vi "Lab Panel V4.82.vi"() -> ()   [LabVIEW 2013] (continued)
                    n1780 = global write "Global 1.vi" "RATE(Hz)"("RATE (Hz)") -> ()
                    n1781 = global write "Global 1.vi" "SAMPLES"("SAMPLES") -> ()
                    n1782 = Index Array(array=w2725, index=6) -> (element=→"LAB04-1 (GRAPH)":dynamicdata)
                    n1783 = Index Array(array=w2725, index=7) -> (element=→"LAB04-2 (GRAPH)":dynamicdata)
                    n1784 = Index Array(array=w2725, index=9) -> (element=→"LAB05-2 (GRAPH)":dynamicdata)
                    n1785 = Index Array(array=w2725, index=8) -> (element=→"LAB05-1 (GRAPH)":dynamicdata)
                    n1786 = Index Array(array=w2725, index=5) -> (element=→"LAB03-2 (GRAPH)":dynamicdata)
                    n1787 = Index Array(array=w2725, index=0) -> (element=→"LAB01-1 (GRAPH)":dynamicdata)
                    n1788 = Index Array(array=w2725, index=1) -> (element=→"LAB01-2 (GRAPH)":dynamicdata)
                    n1789 = Index Array(array=w2725, index=2) -> (element=→"LAB02-1 (GRAPH)":dynamicdata)
                    n1790 = Index Array(array=w2725, index=3) -> (element=→"LAB02-2 (GRAPH)":dynamicdata)
                    n1791 = Index Array(array=w2725, index=4) -> (element=→"LAB03-1 (GRAPH)":dynamicdata)
                    "AI loop time" <- w2726
                    "Analog Error Array" <- w2727
                  }
                  frame #1 {
                    n1792 = Unbundle By Name(w2774) -> ("LAB05-1 (A)"=w2772:dbl, "LAB05-1 (V)"=w2771:dbl, "LAB05-1 (PF)"=w2770:dbl, "LAB05-2 (A)"=w2769:dbl, "LAB05-2 (V)"=w2768:dbl, "LAB05-2 (PF)"=w2767:dbl)
                    n1793 = case shown="False" w2750 {
                      tunnel: [w2775 w2776] -> w2773
                      tunnel: w2749 -> [_ w2776]
                      frame False {
                        n1794 = local read "CAL LAB01"() -> (w2775:T8)
                      }
                      frame True {
                      }
                    }
                    n1795 = Unbundle By Name(w2773) -> ("1  (A) cal"=w2766:dbl, "1 (V) cal"=w2765:dbl, "1 (PF) cal"=w2764:dbl, "2 (A) cal"=w2763:dbl, "2 (V) cal"=w2762:dbl, "2 (PF) cal"=w2761:dbl)  [unwired: 4 out]
                    n1796 = Multiply(x=w2772, y=w2766) -> (x*y=w2759:dbl)
                    n1797 = Multiply(x=w2771, y=w2765) -> (x*y=w2758:dbl)
                    n1798 = Multiply(x=w2770, y=w2764) -> (x*y=w2757:dbl)
                    n1799 = Multiply(x=w2769, y=w2763) -> (x*y=w2753:dbl)
                    n1800 = Multiply(x=w2768, y=w2762) -> (x*y=w2752:dbl)
                    n1801 = Multiply(x=w2767, y=w2761) -> (x*y=w2751:dbl)
                    n1802 = local read "SIG LAB01-1"() -> (w2760:T2)
                    n1803 = local read "SIG LAB01-2"() -> (w2755:T2)
                    n1804 = Bundle By Name(cluster=w2760, "AMPS"=w2759, "VOLTS"=w2758, "PF"=w2757) -> (w2756:T2)
                    n1805 = Bundle By Name(cluster=w2755, "AMPS"=w2753, "VOLTS"=w2752, "PF"=w2751) -> (w2754:T2)
                    n1806 = local write "SIG LAB01-2"(w2754) -> ()
                    n1807 = local write "SIG LAB01-1"(w2756) -> ()
                  }
                  frame #2 {
                    n1808 = Unbundle By Name(w2779) -> ("LAB05-1 (A)"=w2801:dbl, "LAB05-1 (V)"=w2800:dbl, "LAB05-1 (PF)"=w2799:dbl, "LAB05-2 (A)"=w2798:dbl, "LAB05-2 (V)"=w2797:dbl, "LAB05-2 (PF)"=w2796:dbl)
                    n1809 = case shown="True" w2778 {
                      tunnel: [w2803 w2804] -> w2802
                      tunnel: w2777 -> [_ w2804]
                      frame False {
                        n1810 = local read "CAL LAB02"() -> (w2803:T9)
                      }
                      frame True {
                      }
                    }
                    n1811 = Unbundle By Name(w2802) -> ("1  (A) cal"=w2795:dbl, "1 (V) cal"=w2794:dbl, "1 (PF) cal"=w2793:dbl, "2 (A) cal"=w2792:dbl, "2 (V) cal"=w2791:dbl, "2 (PF) cal"=w2790:dbl)  [unwired: 4 out]
                    n1812 = Multiply(x=w2801, y=w2795) -> (x*y=w2788:dbl)
                    n1813 = Multiply(x=w2800, y=w2794) -> (x*y=w2787:dbl)
                    n1814 = Multiply(x=w2799, y=w2793) -> (x*y=w2786:dbl)
                    n1815 = Multiply(x=w2798, y=w2792) -> (x*y=w2782:dbl)
                    n1816 = Multiply(x=w2797, y=w2791) -> (x*y=w2781:dbl)
                    n1817 = Multiply(x=w2796, y=w2790) -> (x*y=w2780:dbl)
                    n1818 = local read "SIG LAB02-1"() -> (w2789:T2)
                    n1819 = local read "SIG LAB02-2"() -> (w2784:T2)
                    n1820 = Bundle By Name(cluster=w2789, "AMPS"=w2788, "VOLTS"=w2787, "PF"=w2786) -> (w2785:T2)
                    n1821 = Bundle By Name(cluster=w2784, "AMPS"=w2782, "VOLTS"=w2781, "PF"=w2780) -> (w2783:T2)
                    n1822 = local write "SIG LAB02-2"(w2783) -> ()
                    n1823 = local write "SIG LAB02-1"(w2785) -> ()
                  }
                  frame #3 {
                    n1824 = Unbundle By Name(w2808) -> ("LAB05-1 (A)"=w2829:dbl, "LAB05-1 (V)"=w2828:dbl, "LAB05-1 (PF)"=w2827:dbl, "LAB05-2 (A)"=w2826:dbl, "LAB05-2 (V)"=w2825:dbl, "LAB05-2 (PF)"=w2824:dbl)
                    n1825 = case shown="True" w2806 {
                      tunnel: [w2831 w2832] -> w2830
                      tunnel: w2805 -> [_ w2832]
                      frame False {
                        n1826 = local read "CAL LAB03"() -> (w2831:T8)
                      }
                      frame True {
                      }
                    }
                    n1827 = Unbundle By Name(w2830) -> ("1  (A) cal"=w2823:dbl, "1 (V) cal"=w2822:dbl, "1 (PF) cal"=w2821:dbl, "2 (A) cal"=w2820:dbl, "2 (V) cal"=w2819:dbl, "2 (PF) cal"=w2818:dbl)  [unwired: 4 out]
                    n1828 = Multiply(x=w2829, y=w2823) -> (x*y=w2816:dbl)
                    n1829 = Multiply(x=w2828, y=w2822) -> (x*y=w2807:dbl)
                    n1830 = Multiply(x=w2827, y=w2821) -> (x*y=w2815:dbl)
                    n1831 = Multiply(x=w2826, y=w2820) -> (x*y=w2811:dbl)
                    n1832 = Multiply(x=w2825, y=w2819) -> (x*y=w2810:dbl)
                    n1833 = Multiply(x=w2824, y=w2818) -> (x*y=w2809:dbl)
                    n1834 = local read "SIG LAB03-1"() -> (w2817:T2)
                    n1835 = local read "SIG LAB03-2"() -> (w2813:T2)
                    n1836 = Bundle By Name(cluster=w2817, "AMPS"=w2816, "VOLTS"=w2807, "PF"=w2815) -> (w2814:T2)
                    n1837 = Bundle By Name(cluster=w2813, "AMPS"=w2811, "VOLTS"=w2810, "PF"=w2809) -> (w2812:T2)
                    n1838 = local write "SIG LAB03-2"(w2812) -> ()
                    n1839 = local write "SIG LAB03-1"(w2814) -> ()
                  }
                  frame #4 {
                    n1840 = Unbundle By Name(w2835) -> ("LAB05-1 (A)"=w2857:dbl, "LAB05-1 (V)"=w2856:dbl, "LAB05-1 (PF)"=w2855:dbl, "LAB05-2 (A)"=w2854:dbl, "LAB05-2 (V)"=w2853:dbl, "LAB05-2 (PF)"=w2852:dbl)
                    n1841 = case shown="False" w2834 {
                      tunnel: [w2859 w2860] -> w2858
                      tunnel: w2833 -> [_ w2860]
                      frame False {
                        n1842 = local read "CAL LAB04"() -> (w2859:T8)
                      }
                      frame True {
                      }
                    }
                    n1843 = Unbundle By Name(w2858) -> ("1  (A) cal"=w2851:dbl, "1 (V) cal"=w2850:dbl, "1 (PF) cal"=w2849:dbl, "2 (A) cal"=w2848:dbl, "2 (V) cal"=w2847:dbl, "2 (PF) cal"=w2846:dbl)  [unwired: 4 out]
                    n1844 = Multiply(x=w2857, y=w2851) -> (x*y=w2844:dbl)
                    n1845 = Multiply(x=w2856, y=w2850) -> (x*y=w2843:dbl)
                    n1846 = Multiply(x=w2855, y=w2849) -> (x*y=w2842:dbl)
                    n1847 = Multiply(x=w2854, y=w2848) -> (x*y=w2838:dbl)
                    n1848 = Multiply(x=w2853, y=w2847) -> (x*y=w2837:dbl)
                    n1849 = Multiply(x=w2852, y=w2846) -> (x*y=w2836:dbl)
                    n1850 = local read "SIG LAB04-1"() -> (w2845:T2)
                    n1851 = local read "SIG LAB04-2"() -> (w2840:T2)
                    n1852 = Bundle By Name(cluster=w2845, "AMPS"=w2844, "VOLTS"=w2843, "PF"=w2842) -> (w2841:T2)
                    n1853 = Bundle By Name(cluster=w2840, "AMPS"=w2838, "VOLTS"=w2837, "PF"=w2836) -> (w2839:T2)
                    n1854 = local write "SIG LAB04-2"(w2839) -> ()
                    n1855 = local write "SIG LAB04-1"(w2841) -> ()
                  }
                  frame #5 {
                    n1856 = Unbundle By Name(w2864) -> ("LAB05-1 (A)"=w2885:dbl, "LAB05-1 (V)"=w2863:dbl, "LAB05-1 (PF)"=w2884:dbl, "LAB05-2 (A)"=w2883:dbl, "LAB05-2 (V)"=w2882:dbl, "LAB05-2 (PF)"=w2881:dbl)
                    n1857 = case shown="False" w2862 {
                      tunnel: [w2887 w2888] -> w2886
                      tunnel: w2861 -> [_ w2888]
                      frame False {
                        n1858 = local read "CAL LAB05"() -> (w2887:T8)
                      }
                      frame True {
                      }
                    }
                    n1859 = Unbundle By Name(w2886) -> ("1  (A) cal"=w2880:dbl, "1 (V) cal"=w2879:dbl, "1 (PF) cal"=w2878:dbl, "2 (A) cal"=w2877:dbl, "2 (V) cal"=w2876:dbl, "2 (PF) cal"=w2875:dbl)  [unwired: 4 out]
                    n1860 = Multiply(x=w2885, y=w2880) -> (x*y=w2873:dbl)
                    n1861 = Multiply(x=w2863, y=w2879) -> (x*y=w2872:dbl)
                    n1862 = Multiply(x=w2884, y=w2878) -> (x*y=w2871:dbl)
                    n1863 = Multiply(x=w2883, y=w2877) -> (x*y=w2867:dbl)
                    n1864 = Multiply(x=w2882, y=w2876) -> (x*y=w2866:dbl)
                    n1865 = Multiply(x=w2881, y=w2875) -> (x*y=w2865:dbl)
                    n1866 = local read "SIG LAB05-1"() -> (w2874:T2)
                    n1867 = local read "SIG LAB05-2"() -> (w2869:T2)
                    n1868 = Bundle By Name(cluster=w2874, "AMPS"=w2873, "VOLTS"=w2872, "PF"=w2871) -> (w2870:T2)
                    n1869 = Bundle By Name(cluster=w2869, "AMPS"=w2867, "VOLTS"=w2866, "PF"=w2865) -> (w2868:T2)
                    n1870 = local write "SIG LAB05-2"(w2868) -> ()
                    n1871 = local write "SIG LAB05-1"(w2870) -> ()
                  }
                }
              }
            }
          }
          frame #12 {
            # "save test data to file"
            n1872 = Get Date/Time In Seconds() -> (seconds since 1Jan1904=w2889:timestamp)
            "File Time Stamp" <- w2889
            n1873 = local read "on loops"() -> (w2908:dbl)
            n1874 = local read "jig cycle"() -> (w2905:dbl)
            n1875 = Format Date/Time String(time format string (%c)="%H:%M%:%S", seconds (now)=w2889) -> (date/time string=w2893:string)  [unwired: 1 in]
            n1876 = Add(x=w2908, y=2) -> (x+y=w2906:dbl)
            n1877 = Build Array(w2893) -> (w2892:string[])
            n1878 = Equal?(x=w2905, y=1) -> (x = y?=w2891:bool)
            n1879 = Equal?(x=w2905, y=w2906) -> (x = y?=w2890:bool)
            n1880 = stacked-sequence {
              tunnel: w2904 -> [w2914 _ _ _ _ _ _ _ _ _]
              tunnel: w2903 -> [_ w2990 _ _ _ _ _ _ _ _]
              tunnel: w2902 -> [_ _ w3070 _ _ _ _ _ _ _]
              tunnel: w2901 -> [_ _ _ w3150 _ _ _ _ _ _]
              tunnel: w2900 -> [_ _ _ _ w3230 _ _ _ _ _]
              tunnel: w2899 -> [_ _ _ _ _ w3310 _ _ _ _]
              tunnel: w2898 -> [_ _ _ _ _ _ w3390 _ _ _]
              tunnel: w2897 -> [_ _ _ _ _ _ _ w3470 _ _]
              tunnel: w2896 -> [_ _ _ _ _ _ _ _ w3550 _]
              tunnel: w2895 -> [_ _ _ _ _ _ _ _ _ w3630]
              tunnel: w2892 -> [w2913 w2994 w3074 w3154 w3234 w3314 w3394 w3474 w3554 w3634]
              tunnel: w2891 -> [w2912 w2993 w3073 w3153 w3233 w3313 w3393 w3473 w3553 w3633]
              tunnel: w2890 -> [w2911 w2992 w3072 w3152 w3232 w3312 w3392 w3472 w3552 w3632]
              tunnel: w2889 -> [w2910 w2991 w3071 w3151 w3231 w3311 w3391 w3471 w3551 w3631]
              frame #0 {
                n1881 = case shown="True" w2914 {
                  tunnel: w2913 -> [_ w2919]
                  tunnel: w2912 -> [_ w2918]
                  tunnel: w2911 -> [_ w2916]
                  tunnel: w2910 -> [_ w2915]
                  frame False {
                  }
                  frame True {
                    n1882 = local read "DISP LAB01-1"() -> (w2920:T4)
                    n1883 = local read "SIG LAB01-1"() -> (w2921:T2)
                    n1884 = local read "ON L01-1"() -> (w2917:cluster{"amps":dbl, "volts":dbl, "pf":dbl})
                    n1885 = Unbundle(w2921) -> ("AMPS"=w2927:dbl, "VOLTS"=w2925:dbl, "PF"=w2924:dbl, "Tmp Live"=w2923:dbl, "Tmp Neut"=w2926:dbl)
                    n1886 = Unbundle(w2920) -> ("CYCLE"=w2922:dbl)  [unwired: 2 out]
                    n1887 = stacked-sequence {
                      tunnel: w2927 -> [w2931 w2950]
                      tunnel: w2926 -> [_ w2949]
                      tunnel: w2925 -> [w2930 w2948]
                      tunnel: w2924 -> [w2929 w2947]
                      tunnel: w2923 -> [_ w2946]
                      tunnel: w2922 -> [_ w2945]
                      tunnel: w2919 -> [_ w2944]
                      tunnel: w2918 -> [w2932 _]
                      tunnel: w2917 -> [w2928 w2942]
                      tunnel: w2916 -> [_ w2943]
                      tunnel: w2915 -> [_ w2938]
                      frame #0 {
                        n1888 = case shown="True" w2932 {
                          tunnel: w2931 -> [_ w2937]
                          tunnel: w2930 -> [_ w2936]
                          tunnel: w2929 -> [_ w2935]
                          tunnel: w2928 -> [_ w2933]
                          frame False {
                          }
                          frame True {
                            n1889 = Bundle(cluster=w2933, "amps"=w2937, "volts"=w2936, "pf"=w2935) -> (w2934:cluster{"amps":dbl, "volts":dbl, "pf":dbl})
                            n1890 = local write "ON L01-1"(w2934) -> ()
                          }
                        }
                      }
                      frame #1 {
                        n1891 = Unbundle(w2942) -> ("amps"=w2941:dbl, "volts"=w2940:dbl, "pf"=w2939:dbl)
                        n1892 = case shown="True" w2943 {
                          tunnel: w2950 -> [_ w2951]
                          tunnel: w2949 -> [_ w2989]
                          tunnel: w2948 -> [_ _]
                          tunnel: w2947 -> [_ _]
                          tunnel: w2946 -> [_ w2988]
                          tunnel: w2945 -> [_ w2987]
                          tunnel: w2944 -> [_ w2955]
                          tunnel: w2941 -> [_ w2952]
                          tunnel: w2940 -> [_ w2984]
                          tunnel: w2939 -> [_ w2983]
                          tunnel: w2938 -> [_ w2953]
                          frame False {
                          }
                          frame True {
                            n1893 = local read "TDMS LAB01-1"() -> (w2986:refnum<k34>)
                            n1894 = Build Array(w2984) -> (w2980:dbl[])
                            n1895 = Build Array(w2983) -> (w2979:dbl[])
                            n1896 = Build Array(w2988) -> (w2978:dbl[])
                            n1897 = Build Array(w2989) -> (w2977:dbl[])
                            n1898 = Build Array(w2952) -> (w2982:dbl[])
                            n1899 = Build Array(w2951) -> (w2981:dbl[])
                            n1900 = Build Array(w2987) -> (w2976:dbl[])
                            n1901 = Build Array("AMPS ON", "AMPS OFF", "VOLTS", "PF", "TEMP Live", "TEMP Neut", "CYCLE") -> (w2960:string[])
                            n1902 = Bundle By Name("Y"=w2982, "t0"=w2953) -> (w2975:waveform(dbl))  [unwired: 1 in]
                            n1903 = Bundle By Name("Y"=w2981, "t0"=w2953) -> (w2974:waveform(dbl))  [unwired: 1 in]
                            n1904 = Bundle By Name("Y"=w2980, "t0"=w2953) -> (w2973:waveform(dbl))  [unwired: 1 in]
                            n1905 = Bundle By Name("Y"=w2979, "t0"=w2953) -> (w2972:waveform(dbl))  [unwired: 1 in]
                            n1906 = Bundle By Name("Y"=w2978, "t0"=w2953) -> (w2971:waveform(dbl))  [unwired: 1 in]
                            n1907 = Bundle By Name("Y"=w2977, "t0"=w2953) -> (w2970:waveform(dbl))  [unwired: 1 in]
                            n1908 = Bundle By Name("Y"=w2976, "t0"=w2953) -> (w2969:waveform(dbl))  [unwired: 1 in]
                            n1909 = Build Array(w2975, w2974, w2973, w2972, w2971, w2970, w2969) -> (w2968:waveform(dbl)[])
                            n1910 = TDMS Write(0:w2986, 5:"TEST VALUES", 7:w2960, 9:w2968) -> (4:w2959:refnum<k34>, 6:w2958:string, 15:w2957:errorcluster)  [unwired: 2 in, 1 out]
                            n1911 = TDMS Write(0:w2959, 5:w2958, 7:"TIME", 9:w2955, 11:w2957) -> (15:w2954:errorcluster)  [unwired: 1 in, 3 out]
                            n1912 = local write "data file error"(w2954) -> ()
                          }
                        }
                      }
                    }
                  }
                }
              }
              frame #1 {
                n1913 = case shown="True" w2990 {
                  tunnel: w2994 -> [_ w2999]
                  tunnel: w2993 -> [_ w2998]
                  tunnel: w2992 -> [_ w2996]
                  tunnel: w2991 -> [_ w2995]
                  frame False {
                  }
                  frame True {
                    n1914 = local read "DISP LAB01-2"() -> (w3000:T4)
                    n1915 = local read "SIG LAB01-2"() -> (w3001:T2)
                    n1916 = local read "ON L01-2"() -> (w2997:cluster{"amps":dbl, "volts":dbl, "pf":dbl})
                    n1917 = Unbundle(w3001) -> ("AMPS"=w3007:dbl, "VOLTS"=w3005:dbl, "PF"=w3004:dbl, "Tmp Live"=w3003:dbl, "Tmp Neut"=w3006:dbl)
                    n1918 = Unbundle(w3000) -> ("CYCLE"=w3002:dbl)  [unwired: 2 out]
                    n1919 = stacked-sequence {
                      tunnel: w3007 -> [w3011 w3030]
                      tunnel: w3006 -> [_ w3029]
                      tunnel: w3005 -> [w3010 w3028]
                      tunnel: w3004 -> [w3009 w3027]
                      tunnel: w3003 -> [_ w3026]
                      tunnel: w3002 -> [_ w3025]
                      tunnel: w2999 -> [_ w3024]
                      tunnel: w2998 -> [w3012 _]
                      tunnel: w2997 -> [w3008 w3022]
                      tunnel: w2996 -> [_ w3023]
                      tunnel: w2995 -> [_ w3018]
                      frame #0 {
                        n1920 = case shown="True" w3012 {
                          tunnel: w3011 -> [_ w3017]
                          tunnel: w3010 -> [_ w3016]
                          tunnel: w3009 -> [_ w3015]
                          tunnel: w3008 -> [_ w3013]
                          frame False {
                          }
                          frame True {
                            n1921 = Bundle(cluster=w3013, "amps"=w3017, "volts"=w3016, "pf"=w3015) -> (w3014:cluster{"amps":dbl, "volts":dbl, "pf":dbl})
                            n1922 = local write "ON L01-2"(w3014) -> ()
                          }
                        }
                      }
                      frame #1 {
                        n1923 = Unbundle(w3022) -> ("amps"=w3021:dbl, "volts"=w3020:dbl, "pf"=w3019:dbl)
                        n1924 = case shown="True" w3023 {
                          tunnel: w3030 -> [_ w3062]
                          tunnel: w3029 -> [_ w3069]
                          tunnel: w3028 -> [_ _]
                          tunnel: w3027 -> [_ _]
                          tunnel: w3026 -> [_ w3068]
                          tunnel: w3025 -> [_ w3067]
                          tunnel: w3024 -> [_ w3032]
                          tunnel: w3021 -> [_ w3064]
                          tunnel: w3020 -> [_ w3063]
                          tunnel: w3019 -> [_ w3061]
                          tunnel: w3018 -> [_ w3053]
                          frame False {
                          }
                          frame True {
                            n1925 = local read "TDMS LAB01-2"() -> (w3066:refnum<k34>)
                            n1926 = Build Array(w3063) -> (w3058:dbl[])
                            n1927 = Build Array(w3061) -> (w3057:dbl[])
                            n1928 = Build Array(w3068) -> (w3056:dbl[])
                            n1929 = Build Array(w3069) -> (w3055:dbl[])
                            n1930 = Build Array(w3064) -> (w3060:dbl[])
                            n1931 = Build Array(w3062) -> (w3059:dbl[])
                            n1932 = Build Array(w3067) -> (w3054:dbl[])
                            n1933 = Build Array("AMPS ON", "AMPS OFF", "VOLTS", "PF", "TEMP Live", "TEMP Neut", "CYCLE") -> (w3037:string[])
                            n1934 = Bundle By Name("Y"=w3060, "t0"=w3053) -> (w3052:waveform(dbl))  [unwired: 1 in]
                            n1935 = Bundle By Name("Y"=w3059, "t0"=w3053) -> (w3051:waveform(dbl))  [unwired: 1 in]
                            n1936 = Bundle By Name("Y"=w3058, "t0"=w3053) -> (w3050:waveform(dbl))  [unwired: 1 in]
                            n1937 = Bundle By Name("Y"=w3057, "t0"=w3053) -> (w3049:waveform(dbl))  [unwired: 1 in]
                            n1938 = Bundle By Name("Y"=w3056, "t0"=w3053) -> (w3048:waveform(dbl))  [unwired: 1 in]
                            n1939 = Bundle By Name("Y"=w3055, "t0"=w3053) -> (w3047:waveform(dbl))  [unwired: 1 in]
                            n1940 = Bundle By Name("Y"=w3054, "t0"=w3053) -> (w3046:waveform(dbl))  [unwired: 1 in]
                            n1941 = Build Array(w3052, w3051, w3050, w3049, w3048, w3047, w3046) -> (w3045:waveform(dbl)[])
                            n1942 = TDMS Write(0:w3066, 5:"TEST VALUES", 7:w3037, 9:w3045) -> (4:w3036:refnum<k34>, 6:w3035:string, 15:w3034:errorcluster)  [unwired: 2 in, 1 out]
                            n1943 = TDMS Write(0:w3036, 5:w3035, 7:"TIME", 9:w3032, 11:w3034) -> (15:w3031:errorcluster)  [unwired: 1 in, 3 out]
                            n1944 = local write "data file error"(w3031) -> ()
                          }
                        }
                      }
                    }
                  }
                }
              }
              frame #2 {
                n1945 = case shown="True" w3070 {
                  tunnel: w3074 -> [_ w3079]
                  tunnel: w3073 -> [_ w3078]
                  tunnel: w3072 -> [_ w3076]
                  tunnel: w3071 -> [_ w3075]
                  frame False {
                  }
                  frame True {
                    n1946 = local read "DISP LAB02-1"() -> (w3080:T4)
                    n1947 = local read "SIG LAB02-1"() -> (w3081:T2)
                    n1948 = local read "ON L02-1"() -> (w3077:cluster{"amps":dbl, "volts":dbl, "pf":dbl})
                    n1949 = Unbundle(w3081) -> ("AMPS"=w3087:dbl, "VOLTS"=w3085:dbl, "PF"=w3084:dbl, "Tmp Live"=w3083:dbl, "Tmp Neut"=w3086:dbl)
                    n1950 = Unbundle(w3080) -> ("CYCLE"=w3082:dbl)  [unwired: 2 out]
                    n1951 = stacked-sequence {
                      tunnel: w3087 -> [w3091 w3110]
                      tunnel: w3086 -> [_ w3109]
                      tunnel: w3085 -> [w3090 w3108]
                      tunnel: w3084 -> [w3089 w3107]
                      tunnel: w3083 -> [_ w3106]
                      tunnel: w3082 -> [_ w3105]
                      tunnel: w3079 -> [_ w3104]
                      tunnel: w3078 -> [w3092 _]
                      tunnel: w3077 -> [w3088 w3102]
                      tunnel: w3076 -> [_ w3103]
                      tunnel: w3075 -> [_ w3098]
                      frame #0 {
                        n1952 = case shown="True" w3092 {
                          tunnel: w3091 -> [_ w3097]
                          tunnel: w3090 -> [_ w3096]
                          tunnel: w3089 -> [_ w3095]
                          tunnel: w3088 -> [_ w3093]
                          frame False {
                          }
                          frame True {
                            n1953 = Bundle(cluster=w3093, "amps"=w3097, "volts"=w3096, "pf"=w3095) -> (w3094:cluster{"amps":dbl, "volts":dbl, "pf":dbl})
                            n1954 = local write "ON L02-1"(w3094) -> ()
                          }
                        }
                      }
                      frame #1 {
                        n1955 = Unbundle(w3102) -> ("amps"=w3101:dbl, "volts"=w3100:dbl, "pf"=w3099:dbl)
                        n1956 = case shown="True" w3103 {
                          tunnel: w3110 -> [_ w3142]
                          tunnel: w3109 -> [_ w3149]
                          tunnel: w3108 -> [_ _]
                          tunnel: w3107 -> [_ _]
                          tunnel: w3106 -> [_ w3148]
                          tunnel: w3105 -> [_ w3147]
                          tunnel: w3104 -> [_ w3112]
                          tunnel: w3101 -> [_ w3144]
                          tunnel: w3100 -> [_ w3143]
                          tunnel: w3099 -> [_ w3141]
                          tunnel: w3098 -> [_ w3133]
                          frame False {
                          }
                          frame True {
                            n1957 = local read "TDMS LAB02-1"() -> (w3146:refnum<k34>)
                            n1958 = Build Array(w3143) -> (w3138:dbl[])
                            n1959 = Build Array(w3141) -> (w3137:dbl[])
                            n1960 = Build Array(w3148) -> (w3136:dbl[])
                            n1961 = Build Array(w3149) -> (w3135:dbl[])
                            n1962 = Build Array(w3144) -> (w3140:dbl[])
                            n1963 = Build Array(w3142) -> (w3139:dbl[])
                            n1964 = Build Array(w3147) -> (w3134:dbl[])
                            n1965 = Build Array("AMPS ON", "AMPS OFF", "VOLTS", "PF", "TEMP Live", "TEMP Neut", "CYCLE") -> (w3117:string[])
                            n1966 = Bundle By Name("Y"=w3140, "t0"=w3133) -> (w3132:waveform(dbl))  [unwired: 1 in]
                            n1967 = Bundle By Name("Y"=w3139, "t0"=w3133) -> (w3131:waveform(dbl))  [unwired: 1 in]
                            n1968 = Bundle By Name("Y"=w3138, "t0"=w3133) -> (w3130:waveform(dbl))  [unwired: 1 in]
                            n1969 = Bundle By Name("Y"=w3137, "t0"=w3133) -> (w3129:waveform(dbl))  [unwired: 1 in]
                            n1970 = Bundle By Name("Y"=w3136, "t0"=w3133) -> (w3128:waveform(dbl))  [unwired: 1 in]
                            n1971 = Bundle By Name("Y"=w3135, "t0"=w3133) -> (w3127:waveform(dbl))  [unwired: 1 in]
                            n1972 = Bundle By Name("Y"=w3134, "t0"=w3133) -> (w3126:waveform(dbl))  [unwired: 1 in]
                            n1973 = Build Array(w3132, w3131, w3130, w3129, w3128, w3127, w3126) -> (w3125:waveform(dbl)[])
                            n1974 = TDMS Write(0:w3146, 5:"TEST VALUES", 7:w3117, 9:w3125) -> (4:w3116:refnum<k34>, 6:w3115:string, 15:w3114:errorcluster)  [unwired: 2 in, 1 out]
                            n1975 = TDMS Write(0:w3116, 5:w3115, 7:"TIME", 9:w3112, 11:w3114) -> (15:w3111:errorcluster)  [unwired: 1 in, 3 out]
                            n1976 = local write "data file error"(w3111) -> ()
                          }
                        }
                      }
                    }
                  }
                }
              }
              frame #3 {
                n1977 = case shown="True" w3150 {
                  tunnel: w3154 -> [_ w3159]
                  tunnel: w3153 -> [_ w3158]
                  tunnel: w3152 -> [_ w3156]
                  tunnel: w3151 -> [_ w3155]
                  frame False {
                  }
                  frame True {
                    n1978 = local read "DISP LAB02-2"() -> (w3160:T4)
                    n1979 = local read "SIG LAB02-2"() -> (w3161:T2)
                    n1980 = local read "ON L02-2"() -> (w3157:cluster{"amps":dbl, "volts":dbl, "pf":dbl})
                    n1981 = Unbundle(w3161) -> ("AMPS"=w3167:dbl, "VOLTS"=w3165:dbl, "PF"=w3164:dbl, "Tmp Live"=w3163:dbl, "Tmp Neut"=w3166:dbl)
                    n1982 = Unbundle(w3160) -> ("CYCLE"=w3162:dbl)  [unwired: 2 out]
                    n1983 = stacked-sequence {
                      tunnel: w3167 -> [w3171 w3190]
                      tunnel: w3166 -> [_ w3189]
                      tunnel: w3165 -> [w3170 w3188]
                      tunnel: w3164 -> [w3169 w3187]
                      tunnel: w3163 -> [_ w3186]
                      tunnel: w3162 -> [_ w3185]
                      tunnel: w3159 -> [_ w3184]
                      tunnel: w3158 -> [w3172 _]
                      tunnel: w3157 -> [w3168 w3182]
                      tunnel: w3156 -> [_ w3183]
                      tunnel: w3155 -> [_ w3178]
                      frame #0 {
                        n1984 = case shown="True" w3172 {
                          tunnel: w3171 -> [_ w3177]
                          tunnel: w3170 -> [_ w3176]
                          tunnel: w3169 -> [_ w3175]
                          tunnel: w3168 -> [_ w3173]
                          frame False {
                          }
                          frame True {
                            n1985 = Bundle(cluster=w3173, "amps"=w3177, "volts"=w3176, "pf"=w3175) -> (w3174:cluster{"amps":dbl, "volts":dbl, "pf":dbl})
                            n1986 = local write "ON L02-2"(w3174) -> ()
                          }
                        }
                      }
                      frame #1 {
                        n1987 = Unbundle(w3182) -> ("amps"=w3181:dbl, "volts"=w3180:dbl, "pf"=w3179:dbl)
                        n1988 = case shown="True" w3183 {
                          tunnel: w3190 -> [_ w3222]
                          tunnel: w3189 -> [_ w3229]
                          tunnel: w3188 -> [_ _]
                          tunnel: w3187 -> [_ _]
                          tunnel: w3186 -> [_ w3228]
                          tunnel: w3185 -> [_ w3227]
                          tunnel: w3184 -> [_ w3192]
                          tunnel: w3181 -> [_ w3224]
                          tunnel: w3180 -> [_ w3223]
                          tunnel: w3179 -> [_ w3221]
                          tunnel: w3178 -> [_ w3213]
                          frame False {
                          }
                          frame True {
                            n1989 = local read "TDMS LAB02-2"() -> (w3226:refnum<k34>)
                            n1990 = Build Array(w3223) -> (w3218:dbl[])
                            n1991 = Build Array(w3221) -> (w3217:dbl[])
                            n1992 = Build Array(w3228) -> (w3216:dbl[])
                            n1993 = Build Array(w3229) -> (w3215:dbl[])
                            n1994 = Build Array(w3224) -> (w3220:dbl[])
                            n1995 = Build Array(w3222) -> (w3219:dbl[])
                            n1996 = Build Array(w3227) -> (w3214:dbl[])
                            n1997 = Build Array("AMPS ON", "AMPS OFF", "VOLTS", "PF", "TEMP Live", "TEMP Neut", "CYCLE") -> (w3197:string[])
                            n1998 = Bundle By Name("Y"=w3220, "t0"=w3213) -> (w3212:waveform(dbl))  [unwired: 1 in]
                            n1999 = Bundle By Name("Y"=w3219, "t0"=w3213) -> (w3211:waveform(dbl))  [unwired: 1 in]
                            n2000 = Bundle By Name("Y"=w3218, "t0"=w3213) -> (w3210:waveform(dbl))  [unwired: 1 in]
                            n2001 = Bundle By Name("Y"=w3217, "t0"=w3213) -> (w3209:waveform(dbl))  [unwired: 1 in]
                            n2002 = Bundle By Name("Y"=w3216, "t0"=w3213) -> (w3208:waveform(dbl))  [unwired: 1 in]
                            n2003 = Bundle By Name("Y"=w3215, "t0"=w3213) -> (w3207:waveform(dbl))  [unwired: 1 in]
                            n2004 = Bundle By Name("Y"=w3214, "t0"=w3213) -> (w3206:waveform(dbl))  [unwired: 1 in]
                            n2005 = Build Array(w3212, w3211, w3210, w3209, w3208, w3207, w3206) -> (w3205:waveform(dbl)[])
                            n2006 = TDMS Write(0:w3226, 5:"TEST VALUES", 7:w3197, 9:w3205) -> (4:w3196:refnum<k34>, 6:w3195:string, 15:w3194:errorcluster)  [unwired: 2 in, 1 out]
                            n2007 = TDMS Write(0:w3196, 5:w3195, 7:"TIME", 9:w3192, 11:w3194) -> (15:w3191:errorcluster)  [unwired: 1 in, 3 out]
                            n2008 = local write "data file error"(w3191) -> ()
                          }
                        }
                      }
                    }
                  }
                }
              }
              frame #4 {
                n2009 = case shown="True" w3230 {
                  tunnel: w3234 -> [_ w3239]
                  tunnel: w3233 -> [_ w3238]
                  tunnel: w3232 -> [_ w3236]
                  tunnel: w3231 -> [_ w3235]
                  frame False {
                  }
                  frame True {
                    n2010 = local read "DISP LAB03-1"() -> (w3240:T4)
                    n2011 = local read "SIG LAB03-1"() -> (w3241:T2)
                    n2012 = local read "ON L03-1"() -> (w3237:cluster{"amps":dbl, "volts":dbl, "pf":dbl})
                    n2013 = Unbundle(w3241) -> ("AMPS"=w3247:dbl, "VOLTS"=w3245:dbl, "PF"=w3244:dbl, "Tmp Live"=w3243:dbl, "Tmp Neut"=w3246:dbl)
                    n2014 = Unbundle(w3240) -> ("CYCLE"=w3242:dbl)  [unwired: 2 out]
                    n2015 = stacked-sequence {
                      tunnel: w3247 -> [w3251 w3270]
                      tunnel: w3246 -> [_ w3269]
                      tunnel: w3245 -> [w3250 w3268]
                      tunnel: w3244 -> [w3249 w3267]
                      tunnel: w3243 -> [_ w3266]
                      tunnel: w3242 -> [_ w3265]
                      tunnel: w3239 -> [_ w3264]
                      tunnel: w3238 -> [w3252 _]
                      tunnel: w3237 -> [w3248 w3262]
                      tunnel: w3236 -> [_ w3263]
                      tunnel: w3235 -> [_ w3258]
                      frame #0 {
                        n2016 = case shown="True" w3252 {
                          tunnel: w3251 -> [_ w3257]
                          tunnel: w3250 -> [_ w3256]
                          tunnel: w3249 -> [_ w3255]
                          tunnel: w3248 -> [_ w3253]
                          frame False {
                          }
                          frame True {
                            n2017 = Bundle(cluster=w3253, "amps"=w3257, "volts"=w3256, "pf"=w3255) -> (w3254:cluster{"amps":dbl, "volts":dbl, "pf":dbl})
                            n2018 = local write "ON L03-1"(w3254) -> ()
                          }
                        }
                      }
                      frame #1 {
                        n2019 = Unbundle(w3262) -> ("amps"=w3261:dbl, "volts"=w3260:dbl, "pf"=w3259:dbl)
                        n2020 = case shown="True" w3263 {
                          tunnel: w3270 -> [_ w3302]
                          tunnel: w3269 -> [_ w3309]
                          tunnel: w3268 -> [_ _]
                          tunnel: w3267 -> [_ _]
                          tunnel: w3266 -> [_ w3308]
                          tunnel: w3265 -> [_ w3307]
                          tunnel: w3264 -> [_ w3272]
                          tunnel: w3261 -> [_ w3304]
                          tunnel: w3260 -> [_ w3303]
                          tunnel: w3259 -> [_ w3301]
                          tunnel: w3258 -> [_ w3293]
                          frame False {
                          }
                          frame True {
                            n2021 = local read "TDMS LAB03-1"() -> (w3306:refnum<k34>)
                            n2022 = Build Array(w3303) -> (w3298:dbl[])
                            n2023 = Build Array(w3301) -> (w3297:dbl[])
                            n2024 = Build Array(w3308) -> (w3296:dbl[])
                            n2025 = Build Array(w3309) -> (w3295:dbl[])
                            n2026 = Build Array(w3304) -> (w3300:dbl[])
                            n2027 = Build Array(w3302) -> (w3299:dbl[])
                            n2028 = Build Array(w3307) -> (w3294:dbl[])
                            n2029 = Build Array("AMPS ON", "AMPS OFF", "VOLTS", "PF", "TEMP Live", "TEMP Neut", "CYCLE") -> (w3277:string[])
                            n2030 = Bundle By Name("Y"=w3300, "t0"=w3293) -> (w3292:waveform(dbl))  [unwired: 1 in]
                            n2031 = Bundle By Name("Y"=w3299, "t0"=w3293) -> (w3291:waveform(dbl))  [unwired: 1 in]
                            n2032 = Bundle By Name("Y"=w3298, "t0"=w3293) -> (w3290:waveform(dbl))  [unwired: 1 in]
                            n2033 = Bundle By Name("Y"=w3297, "t0"=w3293) -> (w3289:waveform(dbl))  [unwired: 1 in]
                            n2034 = Bundle By Name("Y"=w3296, "t0"=w3293) -> (w3288:waveform(dbl))  [unwired: 1 in]
                            n2035 = Bundle By Name("Y"=w3295, "t0"=w3293) -> (w3287:waveform(dbl))  [unwired: 1 in]
                            n2036 = Bundle By Name("Y"=w3294, "t0"=w3293) -> (w3286:waveform(dbl))  [unwired: 1 in]
                            n2037 = Build Array(w3292, w3291, w3290, w3289, w3288, w3287, w3286) -> (w3285:waveform(dbl)[])
                            n2038 = TDMS Write(0:w3306, 5:"TEST VALUES", 7:w3277, 9:w3285) -> (4:w3276:refnum<k34>, 6:w3275:string, 15:w3274:errorcluster)  [unwired: 2 in, 1 out]
                            n2039 = TDMS Write(0:w3276, 5:w3275, 7:"TIME", 9:w3272, 11:w3274) -> (15:w3271:errorcluster)  [unwired: 1 in, 3 out]
                            n2040 = local write "data file error"(w3271) -> ()
                          }
                        }
                      }
                    }
                  }
                }
              }
              frame #5 {
                n2041 = case shown="True" w3310 {
                  tunnel: w3314 -> [_ w3319]
                  tunnel: w3313 -> [_ w3318]
                  tunnel: w3312 -> [_ w3316]
                  tunnel: w3311 -> [_ w3315]
                  frame False {
                  }
                  frame True {
                    n2042 = local read "DISP LAB03-2"() -> (w3320:T4)
                    n2043 = local read "SIG LAB03-2"() -> (w3321:T2)
                    n2044 = local read "ON L03-2"() -> (w3317:cluster{"amps":dbl, "volts":dbl, "pf":dbl})
                    n2045 = Unbundle(w3321) -> ("AMPS"=w3327:dbl, "VOLTS"=w3325:dbl, "PF"=w3324:dbl, "Tmp Live"=w3323:dbl, "Tmp Neut"=w3326:dbl)
                    n2046 = Unbundle(w3320) -> ("CYCLE"=w3322:dbl)  [unwired: 2 out]
                    n2047 = stacked-sequence {
                      tunnel: w3327 -> [w3331 w3350]
                      tunnel: w3326 -> [_ w3349]
                      tunnel: w3325 -> [w3330 w3348]
                      tunnel: w3324 -> [w3329 w3347]
                      tunnel: w3323 -> [_ w3346]
                      tunnel: w3322 -> [_ w3345]
                      tunnel: w3319 -> [_ w3344]
                      tunnel: w3318 -> [w3332 _]
                      tunnel: w3317 -> [w3328 w3342]
                      tunnel: w3316 -> [_ w3343]
                      tunnel: w3315 -> [_ w3338]
                      frame #0 {
                        n2048 = case shown="True" w3332 {
                          tunnel: w3331 -> [_ w3337]
                          tunnel: w3330 -> [_ w3336]
                          tunnel: w3329 -> [_ w3335]
                          tunnel: w3328 -> [_ w3333]
                          frame False {
                          }
                          frame True {
                            n2049 = Bundle(cluster=w3333, "amps"=w3337, "volts"=w3336, "pf"=w3335) -> (w3334:cluster{"amps":dbl, "volts":dbl, "pf":dbl})
                            n2050 = local write "ON L03-2"(w3334) -> ()
                          }
                        }
                      }
                      frame #1 {
                        n2051 = Unbundle(w3342) -> ("amps"=w3341:dbl, "volts"=w3340:dbl, "pf"=w3339:dbl)
                        n2052 = case shown="True" w3343 {
                          tunnel: w3350 -> [_ w3382]
                          tunnel: w3349 -> [_ w3389]
                          tunnel: w3348 -> [_ _]
                          tunnel: w3347 -> [_ _]
                          tunnel: w3346 -> [_ w3388]
                          tunnel: w3345 -> [_ w3387]
                          tunnel: w3344 -> [_ w3352]
                          tunnel: w3341 -> [_ w3384]
                          tunnel: w3340 -> [_ w3383]
                          tunnel: w3339 -> [_ w3381]
                          tunnel: w3338 -> [_ w3373]
                          frame False {
                          }
                          frame True {
                            n2053 = local read "TDMS LAB03-2"() -> (w3386:refnum<k34>)
                            n2054 = Build Array(w3383) -> (w3378:dbl[])
                            n2055 = Build Array(w3381) -> (w3377:dbl[])
                            n2056 = Build Array(w3388) -> (w3376:dbl[])
                            n2057 = Build Array(w3389) -> (w3375:dbl[])
                            n2058 = Build Array(w3384) -> (w3380:dbl[])
                            n2059 = Build Array(w3382) -> (w3379:dbl[])
                            n2060 = Build Array(w3387) -> (w3374:dbl[])
                            n2061 = Build Array("AMPS ON", "AMPS OFF", "VOLTS", "PF", "TEMP Live", "TEMP Neut", "CYCLE") -> (w3357:string[])
                            n2062 = Bundle By Name("Y"=w3380, "t0"=w3373) -> (w3372:waveform(dbl))  [unwired: 1 in]
                            n2063 = Bundle By Name("Y"=w3379, "t0"=w3373) -> (w3371:waveform(dbl))  [unwired: 1 in]
                            n2064 = Bundle By Name("Y"=w3378, "t0"=w3373) -> (w3370:waveform(dbl))  [unwired: 1 in]
                            n2065 = Bundle By Name("Y"=w3377, "t0"=w3373) -> (w3369:waveform(dbl))  [unwired: 1 in]
                            n2066 = Bundle By Name("Y"=w3376, "t0"=w3373) -> (w3368:waveform(dbl))  [unwired: 1 in]
                            n2067 = Bundle By Name("Y"=w3375, "t0"=w3373) -> (w3367:waveform(dbl))  [unwired: 1 in]
                            n2068 = Bundle By Name("Y"=w3374, "t0"=w3373) -> (w3366:waveform(dbl))  [unwired: 1 in]
                            n2069 = Build Array(w3372, w3371, w3370, w3369, w3368, w3367, w3366) -> (w3365:waveform(dbl)[])
                            n2070 = TDMS Write(0:w3386, 5:"TEST VALUES", 7:w3357, 9:w3365) -> (4:w3356:refnum<k34>, 6:w3355:string, 15:w3354:errorcluster)  [unwired: 2 in, 1 out]
                            n2071 = TDMS Write(0:w3356, 5:w3355, 7:"TIME", 9:w3352, 11:w3354) -> (15:w3351:errorcluster)  [unwired: 1 in, 3 out]
                            n2072 = local write "data file error"(w3351) -> ()
                          }
                        }
                      }
                    }
                  }
                }
              }
              frame #6 {
                n2073 = case shown="True" w3390 {
                  tunnel: w3394 -> [_ w3399]
                  tunnel: w3393 -> [_ w3398]
                  tunnel: w3392 -> [_ w3396]
                  tunnel: w3391 -> [_ w3395]
                  frame False {
                  }
                  frame True {
                    n2074 = local read "DISP LAB04-1"() -> (w3400:T4)
                    n2075 = local read "SIG LAB04-1"() -> (w3401:T2)
                    n2076 = local read "ON L04-1"() -> (w3397:cluster{"amps":dbl, "volts":dbl, "pf":dbl})
                    n2077 = Unbundle(w3401) -> ("AMPS"=w3407:dbl, "VOLTS"=w3405:dbl, "PF"=w3404:dbl, "Tmp Live"=w3403:dbl, "Tmp Neut"=w3406:dbl)
                    n2078 = Unbundle(w3400) -> ("CYCLE"=w3402:dbl)  [unwired: 2 out]
                    n2079 = stacked-sequence {
                      tunnel: w3407 -> [w3411 w3430]
                      tunnel: w3406 -> [_ w3429]
                      tunnel: w3405 -> [w3410 w3428]
                      tunnel: w3404 -> [w3409 w3427]
                      tunnel: w3403 -> [_ w3426]
                      tunnel: w3402 -> [_ w3425]
                      tunnel: w3399 -> [_ w3424]
                      tunnel: w3398 -> [w3412 _]
                      tunnel: w3397 -> [w3408 w3422]
                      tunnel: w3396 -> [_ w3423]
                      tunnel: w3395 -> [_ w3418]
                      frame #0 {
                        n2080 = case shown="True" w3412 {
                          tunnel: w3411 -> [_ w3417]
                          tunnel: w3410 -> [_ w3416]
                          tunnel: w3409 -> [_ w3415]
                          tunnel: w3408 -> [_ w3413]
                          frame False {
                          }
                          frame True {
                            n2081 = Bundle(cluster=w3413, "amps"=w3417, "volts"=w3416, "pf"=w3415) -> (w3414:cluster{"amps":dbl, "volts":dbl, "pf":dbl})
                            n2082 = local write "ON L04-1"(w3414) -> ()
                          }
                        }
                      }
                      frame #1 {
                        n2083 = Unbundle(w3422) -> ("amps"=w3421:dbl, "volts"=w3420:dbl, "pf"=w3419:dbl)
                        n2084 = case shown="True" w3423 {
                          tunnel: w3430 -> [_ w3462]
                          tunnel: w3429 -> [_ w3469]
                          tunnel: w3428 -> [_ _]
                          tunnel: w3427 -> [_ _]
                          tunnel: w3426 -> [_ w3468]
                          tunnel: w3425 -> [_ w3467]
                          tunnel: w3424 -> [_ w3432]
                          tunnel: w3421 -> [_ w3464]
                          tunnel: w3420 -> [_ w3463]
                          tunnel: w3419 -> [_ w3461]
                          tunnel: w3418 -> [_ w3453]
                          frame False {
                          }
                          frame True {
                            n2085 = local read "TDMS LAB04-1"() -> (w3466:refnum<k34>)
                            n2086 = Build Array(w3463) -> (w3458:dbl[])
                            n2087 = Build Array(w3461) -> (w3457:dbl[])
                            n2088 = Build Array(w3468) -> (w3456:dbl[])
                            n2089 = Build Array(w3469) -> (w3455:dbl[])
                            n2090 = Build Array(w3464) -> (w3460:dbl[])
                            n2091 = Build Array(w3462) -> (w3459:dbl[])
                            n2092 = Build Array(w3467) -> (w3454:dbl[])
                            n2093 = Build Array("AMPS ON", "AMPS OFF", "VOLTS", "PF", "TEMP Live", "TEMP Neut", "CYCLE") -> (w3437:string[])
                            n2094 = Bundle By Name("Y"=w3460, "t0"=w3453) -> (w3452:waveform(dbl))  [unwired: 1 in]
                            n2095 = Bundle By Name("Y"=w3459, "t0"=w3453) -> (w3451:waveform(dbl))  [unwired: 1 in]
                            n2096 = Bundle By Name("Y"=w3458, "t0"=w3453) -> (w3450:waveform(dbl))  [unwired: 1 in]
                            n2097 = Bundle By Name("Y"=w3457, "t0"=w3453) -> (w3449:waveform(dbl))  [unwired: 1 in]
                            n2098 = Bundle By Name("Y"=w3456, "t0"=w3453) -> (w3448:waveform(dbl))  [unwired: 1 in]
                            n2099 = Bundle By Name("Y"=w3455, "t0"=w3453) -> (w3447:waveform(dbl))  [unwired: 1 in]
                            n2100 = Bundle By Name("Y"=w3454, "t0"=w3453) -> (w3446:waveform(dbl))  [unwired: 1 in]
                            n2101 = Build Array(w3452, w3451, w3450, w3449, w3448, w3447, w3446) -> (w3445:waveform(dbl)[])
                            n2102 = TDMS Write(0:w3466, 5:"TEST VALUES", 7:w3437, 9:w3445) -> (4:w3436:refnum<k34>, 6:w3435:string, 15:w3434:errorcluster)  [unwired: 2 in, 1 out]
                            n2103 = TDMS Write(0:w3436, 5:w3435, 7:"TIME", 9:w3432, 11:w3434) -> (15:w3431:errorcluster)  [unwired: 1 in, 3 out]
                            n2104 = local write "data file error"(w3431) -> ()
                          }
                        }
                      }
                    }
                  }
                }
              }
              frame #7 {
                n2105 = case shown="True" w3470 {
                  tunnel: w3474 -> [_ w3479]
                  tunnel: w3473 -> [_ w3478]
                  tunnel: w3472 -> [_ w3476]
                  tunnel: w3471 -> [_ w3475]
                  frame False {
                  }
                  frame True {
                    n2106 = local read "DISP LAB04-2"() -> (w3480:T4)
                    n2107 = local read "SIG LAB04-2"() -> (w3481:T2)
                    n2108 = local read "ON L04-2"() -> (w3477:cluster{"amps":dbl, "volts":dbl, "pf":dbl})
                    n2109 = Unbundle(w3481) -> ("AMPS"=w3487:dbl, "VOLTS"=w3485:dbl, "PF"=w3484:dbl, "Tmp Live"=w3483:dbl, "Tmp Neut"=w3486:dbl)
                    n2110 = Unbundle(w3480) -> ("CYCLE"=w3482:dbl)  [unwired: 2 out]
                    n2111 = stacked-sequence {
                      tunnel: w3487 -> [w3491 w3510]
                      tunnel: w3486 -> [_ w3509]
                      tunnel: w3485 -> [w3490 w3508]
                      tunnel: w3484 -> [w3489 w3507]
                      tunnel: w3483 -> [_ w3506]
                      tunnel: w3482 -> [_ w3505]
                      tunnel: w3479 -> [_ w3504]
                      tunnel: w3478 -> [w3492 _]
                      tunnel: w3477 -> [w3488 w3502]
                      tunnel: w3476 -> [_ w3503]
                      tunnel: w3475 -> [_ w3498]
                      frame #0 {
                        n2112 = case shown="True" w3492 {
                          tunnel: w3491 -> [_ w3497]
                          tunnel: w3490 -> [_ w3496]
                          tunnel: w3489 -> [_ w3495]
                          tunnel: w3488 -> [_ w3493]
                          frame False {
                          }
                          frame True {
                            n2113 = Bundle(cluster=w3493, "amps"=w3497, "volts"=w3496, "pf"=w3495) -> (w3494:cluster{"amps":dbl, "volts":dbl, "pf":dbl})
